vi "Do.vi"(8 "error in (no error)":errorcluster, 10 "Actor in":refnum<class "Actor.lvclass">, 11 "Register Create Test Channel Sensor Names Msg in":refnum<class "Register Create Test Channel Sensor Names Msg.lvclass">) -> (0 "error out":errorcluster, 2 "Actor out":refnum<class "Actor.lvclass">)   [LabVIEW 2013, in "Create Test Channel Model.lvlib" / "Register Create Test Channel Sensor Names Msg.lvclass"]
doc: "(<B>Filename</B>: Actor Framework.lvlib:Message.lvclass:Do.vi)\n\nDefines what a message does when it is received by an actor. Generally, a message instructs an actor to invoke one of its methods.\n\nBy default, this method does nothing. A child class must override it to define behavior. Create a child class by using the Actor Framework Message Maker dialog box."
uses:
  Register Create Test Channel Sensor Names Msg.lvclass
  <vilib>/ActorFramework/Actor/Actor.lvclass
  Create Test Channel Model/Create Test Channel Model.lvclass
  <vilib>/ActorFrameworkMVC/View Observer/Registration Message/Registration Message.lvclass/Registration Message.ctl
  <vilib>/ActorFramework/Message Enqueuer/Message Enqueuer.lvclass
  <vilib>/ActorFrameworkMVC/View Observer/Data Message/Data Message.lvclass
  <vilib>/ActorFrameworkMVC/View Observer/Registration Message/Registration Message.lvclass
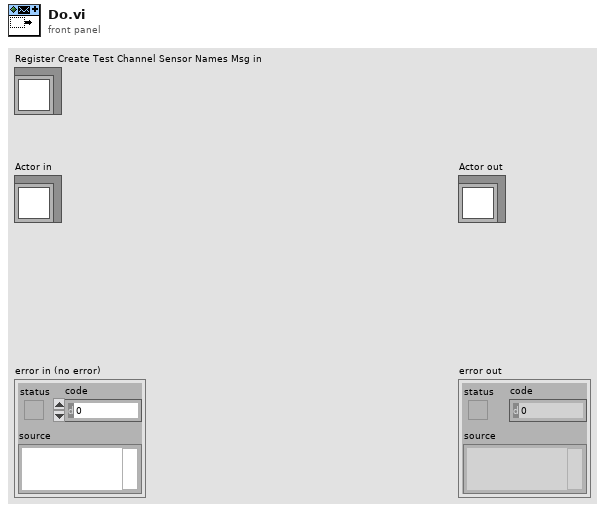
[diagram p1: front panel]
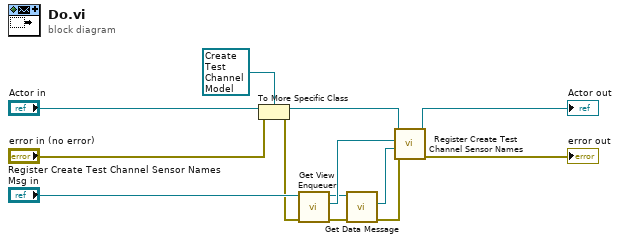
[diagram p0: block diagram]
diagram:
  n1 = To More Specific Class(target class=refnum<class "Create Test Channel Model.lvclass"> refnum ("Create Test Channel Model.lvlib:Create Test Channel Model.lvclass"), reference="Actor in", error in="error in (no error)") -> (specific class reference=w4:refnum<class "Create Test Channel Model.lvclass">, error out=w1:errorcluster)
  n2 = call <vilib>:"Get View Enqueuer.vi"("error in (no error)"=w1, "Registration Message in"="Register Create Test Channel Sensor Names Msg in") -> ("error out"=w2:errorcluster, "View Enqueuer"=w9:refnum<class "Message Enqueuer.lvclass">, "Registration Message out"=w7:refnum<class "Register Create Test Channel Sensor Names Msg.lvclass">)  [unwired: 7 in]
  n3 = call <vilib>:"Get Data Message.vi"("error in (no error)"=w2, "Registration Message in"=w7) -> ("error out"=w3:errorcluster, "Data Message"=w8:refnum<class "Data Message.lvclass">)  [unwired: 7 in, 1 out]
  n4 = call "Register Create Test Channel Sensor Names.vi"("error in (no error)"=w3, "Data Message"=w8, "View Enqueuer"=w9, "Create Test Channel Model in"=w4) -> ("error out"=→"error out":errorcluster, "Create Test Channel Model out"=→"Actor out":refnum<class "Create Test Channel Model.lvclass">)  [unwired: 6 in]
